vi "rqcBob Trigger Router (FPGA).vi"(0 "sw":bool, 2 "rqcBob Trigger Type":T1=enum."immediate", 7 "hw":bool) -> (6 "trigger out":bool)   [LabVIEW 2018]
uses:
  Custom Controls/rqcBob Trigger Type.ctl
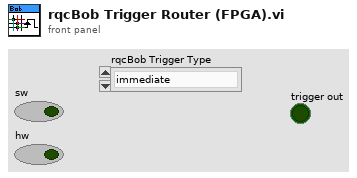
[diagram p1: front panel]
types:
  T1 = typedef "rqcBob Trigger Type.ctl" = enum16{"software", "immediate", "DIO"}
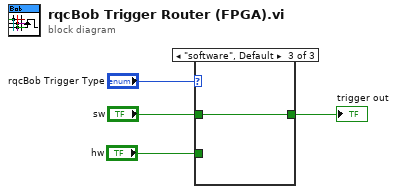
[diagram p0: block diagram]
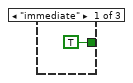
[diagram p2: hidden frame]
diagram:
  n1 = case shown="\"software\", Default" "rqcBob Trigger Type" {
    tunnel: "hw" -> [_ w6 _]
    tunnel: [TRUE ("hw") w6 w7] -> w2
    tunnel: "sw" -> [_ _ w7]
    frame "immediate" {
    }
    frame "DIO" {
    }
    frame "software", Default {
    }
  }
  "trigger out" <- w2
